vi "test.vi"() -> ()   [LabVIEW 2017]
uses:
  Detailed Report/Controls/Detailed_Reports_Columns.ctl
  SQL/SQL/SQL_DB-Enum.ctl
  <vilib>/Utility/error.llb/whitespace.ctl
  <vilib>/addons/database/Auxilliary.llb/DB Tools Column Info.ctl
  <vilib>/addons/database/Auxilliary.llb/DB Tools DataTypes.ctl
  <vilib>/addons/database/NI_Database_API.lvlib
panel:
  out "variant 2":variant
  out "variant":variant
  out "Column Names":T1=["Barcode", "[Date&Time]", "[User Name]", "Shift", "Model", "Variant", "[Test Name]", "[Test Type]", "[Excepted Value]", "HL", "LL", "[Obtained Value]", "Result", "[Cycle Time]", "[NIP Code]"]
  out "error in (no error) 4":errorcluster
  in  "error in (no error) 3":errorcluster
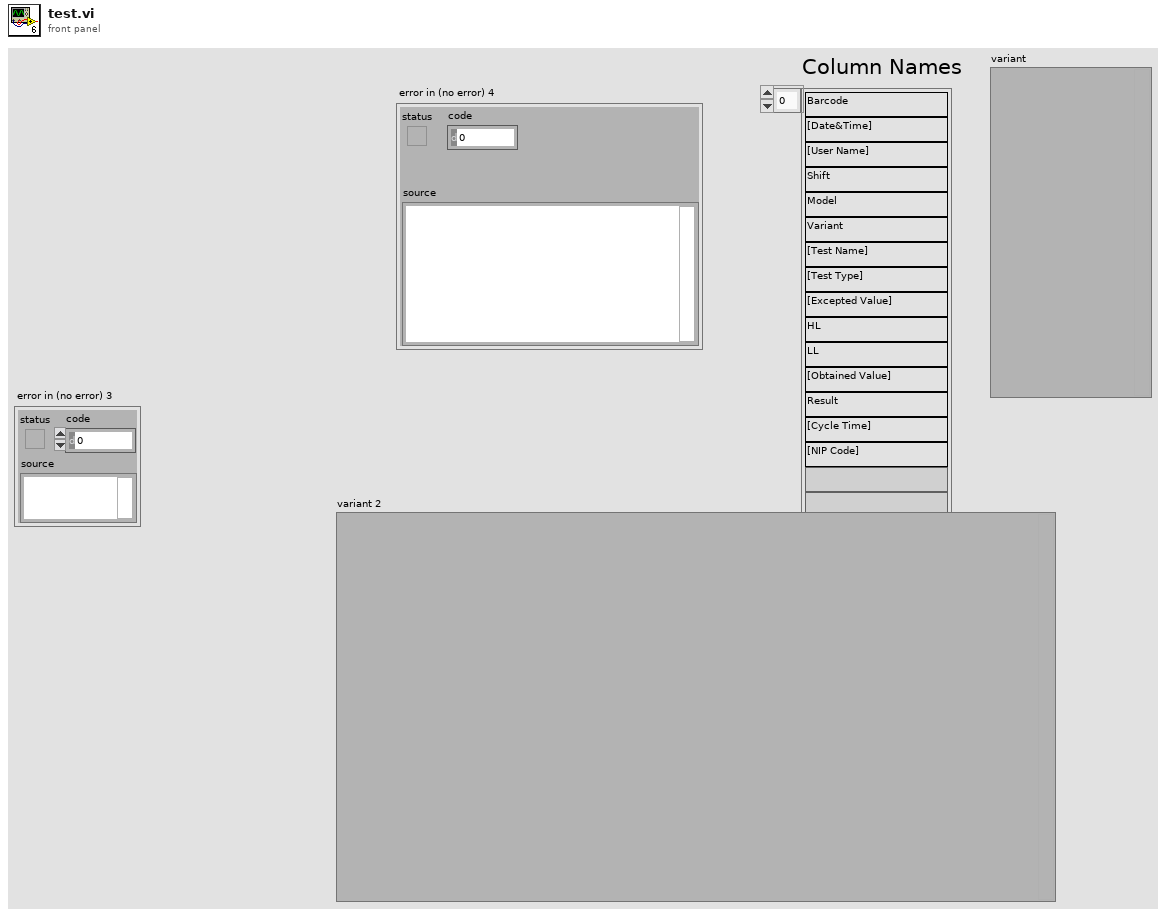
[diagram p1: front panel]
types:
  T1 = typedef "Detailed_Reports_Columns.ctl" = string[]
  T2 = typedef "NI_Database_API.lvlib/DB Tools Column Info.ctl" = cluster{"column name":string, "data type":T3, "size":i32, "allow null?":bool}
  T3 = typedef "NI_Database_API.lvlib/DB Tools DataTypes.ctl" = enum16{"String", "Long (I32)", "Single (SGL)", "Double (DBL)", "Date/Time", "Binary"}
  T4 = typedef "SQL_DB-Enum.ctl" = enum16{"INI DATA", "Open Connections", "Query", "Update Table", "Get Full Report", "Get Serial Numbers", "Get Table Columns", "Get Table Names", "Check & Create Table", "Close Connection"}
  T5 = cluster{string, string, string, string, string, string, string, string, string, string, string, string, string, string, string}
  T6 = typedef "whitespace.ctl" = u16
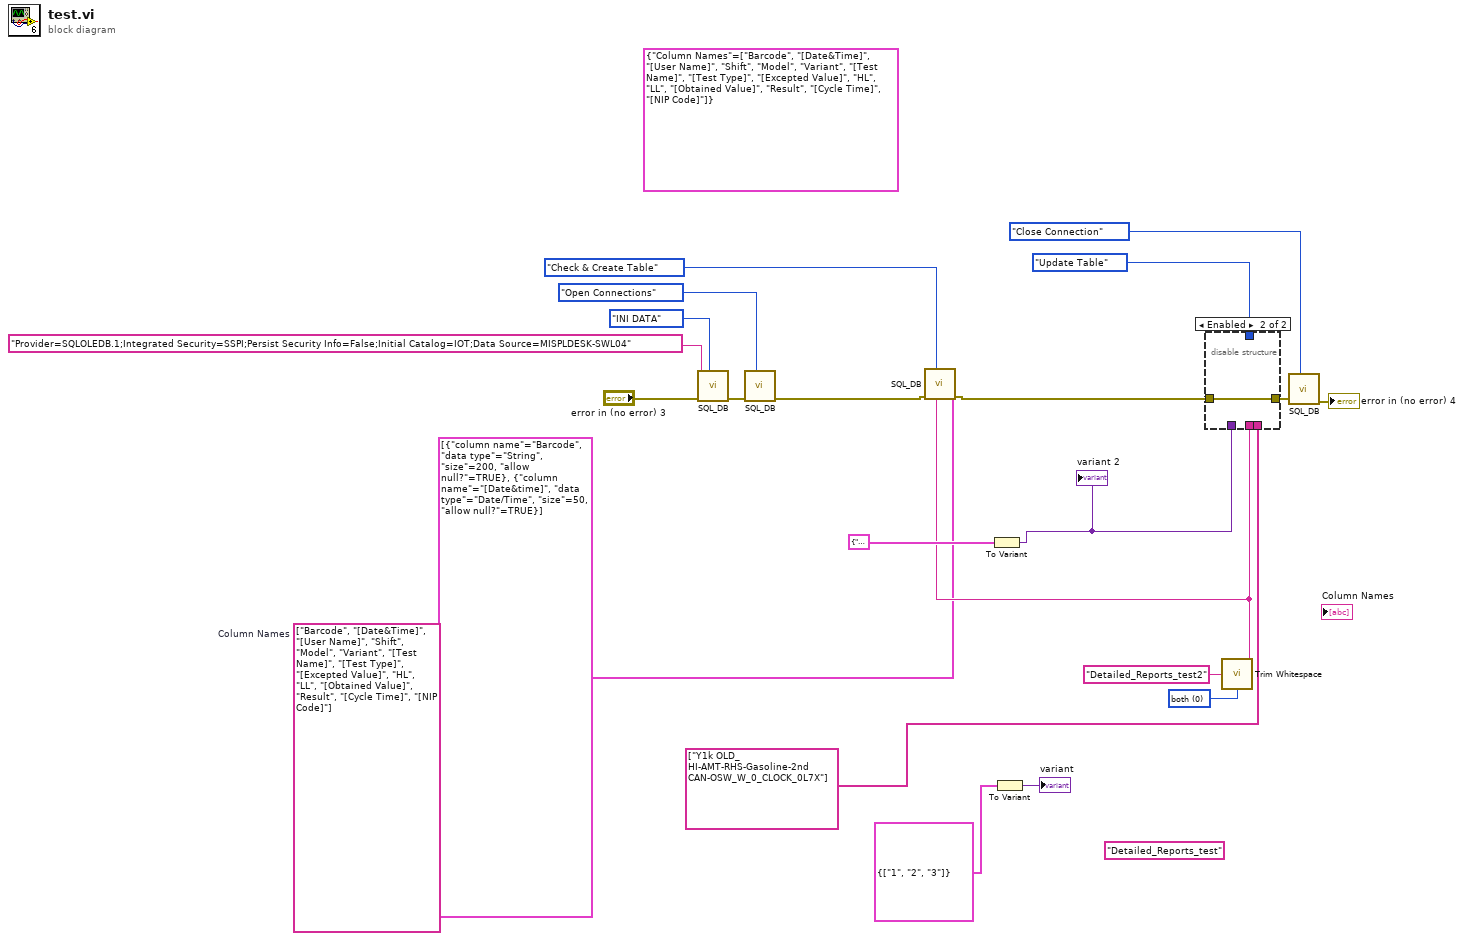
[diagram p0: block diagram]
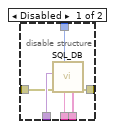
[diagram p2: hidden frame]
diagram:
  (unwired) "Detailed_Reports_test" ("Table Name")
  (unwired) T1 ["Barcode", "[Date&Time]", "[User Name]", "Shift", "Model", "Variant", "[Test Name]", "[Test Type]", "[Excepted Value]", "HL", "LL", "[Obtained Value]", "Result", "[Cycle Time]", "[NIP Code]"]  # Column Names
  (unwired) cluster{"Column Names":T1} {"Column Names"=["Barcode", "[Date&Time]", "[User Name]", "Shift", "Model", "Variant", "[Test Name]", "[Test Type]", "[Excepted Value]", "HL", "LL", "[Obtained Value]", "Result", "[Cycle Time]", "[NIP Code]"]}
  w14 = T6 0 items=["both", "start of string", "end of string"] ("location (both)")
  n1 = call "SQL_DB.vi"("CTRL"=SQL_DB-Enum."INI DATA", "error in (no error)"="error in (no error) 3", "Connection Info"="Provider=SQLOLEDB.1;Integrated Security=SSPI;Persist Security Info=False;Initial Catalog=IOT;Data Source=MISPLDESK-SWL04") -> ("error in (no error) 2"=w21:errorcluster)  [unwired: 6 in, 2 out]
  n2 = call "SQL_DB.vi"("CTRL"=SQL_DB-Enum."Open Connections", "error in (no error)"=w21) -> ("error in (no error) 2"=w6:errorcluster)  [unwired: 7 in, 2 out]
  n3 = To Variant(anything=T5 {"barcode", "2019-12-13 20:24:09.05", "1", "shifr", "model", "variant", "test name", "test type", "hl", "ll", "shifr", "obtained", "resrut", "Cycle time", "nip code"}) -> (Variant=w10:variant)
  "variant 2" <- w10
  n4 = To Variant(anything=cluster{string[]} {["1", "2", "3"]}) -> (Variant=→"variant":variant)
  n5 = call <vilib>:"Trim Whitespace.vi"("string"="Detailed_Reports_test2" ("Table Name"), "location (both)"=w14) -> ("trimmed string"=w3:string)
  n6 = call "SQL_DB.vi"("column information"=T2[] [{"column name"="Barcode", "data type"=enum."String", "size"=200, "allow null?"=TRUE}, {"column name"="[Date&time]", "data type"=enum."Date/Time", "size"=50, "allow null?"=TRUE}], "Table Name"=w3, "CTRL"=SQL_DB-Enum."Check & Create Table", "error in (no error)"=w6) -> ("error in (no error) 2"=w5:errorcluster)  [unwired: 5 in, 2 out]
  n7 = disable-structure shown="Enabled" {
    disable-tunnel: SQL_DB-Enum."Update Table" ("CTRL") -> [w27 _]
    disable-tunnel: [w26 w28] -> w12
    disable-tunnel: w10 -> [w25 _]
    disable-tunnel: w5 -> [w24 w28]
    disable-tunnel: w3 -> [w23 _]
    disable-tunnel: string[] ["Y1k OLD_HI-AMT-RHS-Gasoline-2nd CAN-OSW_W_0_CLOCK_0L7X"] -> [w22 _]
    frame Disabled {
      n8 = call "SQL_DB.vi"("Column Names"=w22, "Table Name"=w23, "CTRL"=w27, "error in (no error)"=w24, "data to Update"=w25) -> ("error in (no error) 2"=w26:errorcluster)  [unwired: 4 in, 2 out]
    }
    frame Enabled {
    }
  }
  n9 = call "SQL_DB.vi"("CTRL"=SQL_DB-Enum."Close Connection", "error in (no error)"=w12) -> ("error in (no error) 2"=→"error in (no error) 4":errorcluster)  [unwired: 7 in, 2 out]
